vi "Pi_Python_REPL.vi"(11 "Pi IP Address":string="130.64.218.232") -> ()   [LabVIEW 2019]
panel:
  in  "Ctrl C":bool
  in  "Script":string="from pybricks import ev3brick as brick\nfrom pybricks.ev3devices import Motor, TouchSensor, ColorSensor,InfraredSensor, UltrasonicSensor, GyroSensor\n\nfrom pybricks.parameters import Port, Stop, Direction, Button, Color, Align\n\nfrom pybricks.tools import wait, StopWatch\n\nexample_motor = Motor (Port.A)"
  out "Console":string
  in  "Help Button":bool
  in  "Run DIrect":bool
  in  "Password":string="buddha"
  in  "Username":string="pi"
  out "SSH Success?":bool
  in  "Done":bool
  # "Get Labview running\n7. pip install paramiko  (SSH)\n8. Run this program\n9. hit ping to make sure it is there\n10. hit SSH In\n11. start python"
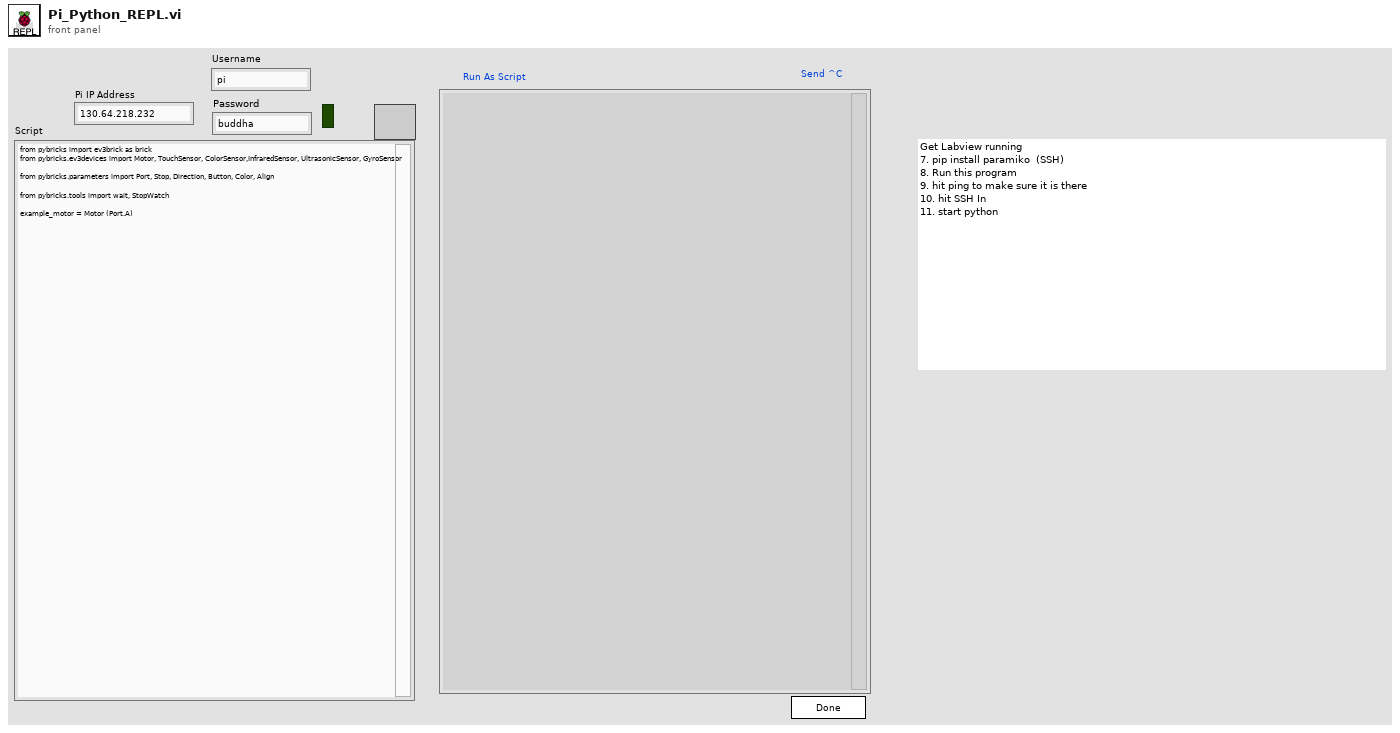
[diagram p1: front panel]
types:
  T1 = typedef "eventvkey.ctl" = enum16{"ASCII", "Enter", "Return", "Shift", "Ctrl", "Alt", "Cmd", "Opt", "Caps", "NumLock", "Clear", "Break", "Up", "Down", "Left", "Right", "Insert", "Delete", "Home", "End", "PageUp", "PageDown", "Escape", "Help", "Pause", "ScrollLock", "F1", "F2", "F3", "F4", "F5", "F6", "F7", "F8", "F9", "F10", "F11", "F12", "F13", "F14", "F15", "F16", "F17", "F18", "F19", "F20", "F21", "F22", "F23", "F24", "Play", "VolumeUp", "VolumeDown", "Mute", "Two Byte Char"}
  T2 = cluster{"Shift":bool, "Ctrl":bool, "Alt":bool, "Cmd":bool, "Opt":bool}
  T3 = cluster{"Char":i16, "VKey":T1, "ScanCode":i16, "Mods":cluster{"Num Pad":bool, "Menu Key":bool}, "PlatMods":cluster{"Shift":bool, "Ctrl":bool, "Alt":bool, "Cmd":bool, "Opt":bool}, "FocusObj":refnum<vi>}
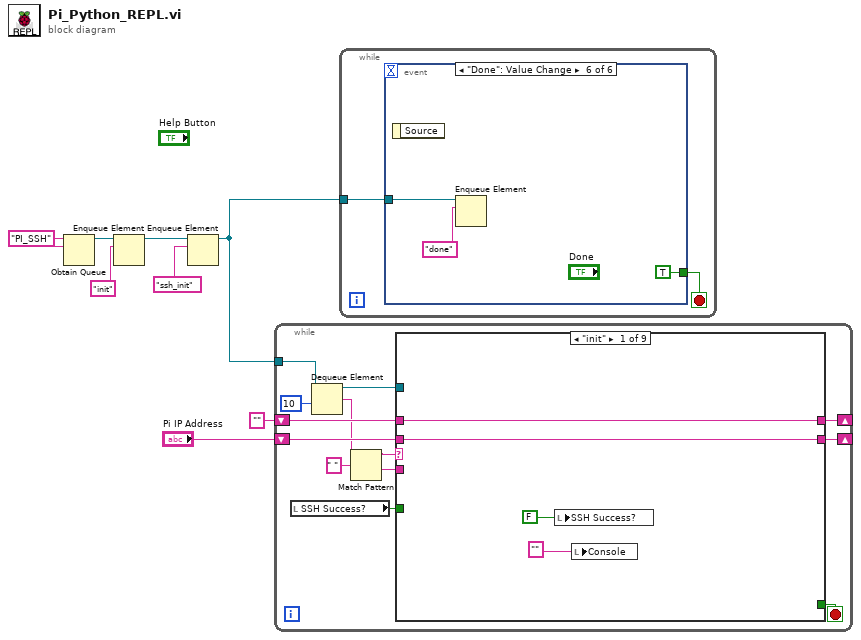
[diagram p0: block diagram]
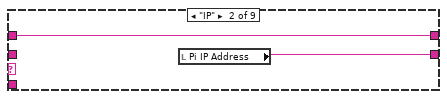
[diagram p2: hidden frame]
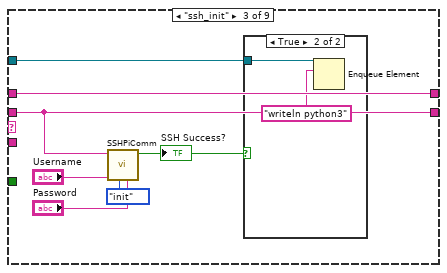
[diagram p3: hidden frame]
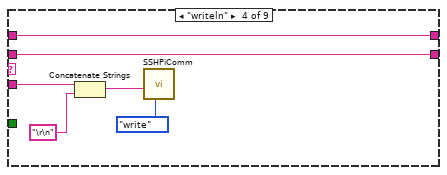
[diagram p5: hidden frame]
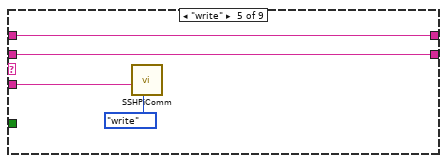
[diagram p6: hidden frame]
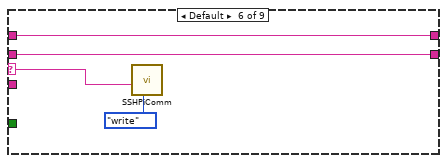
[diagram p7: hidden frame]
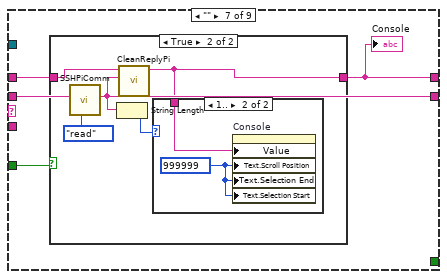
[diagram p8: hidden frame]
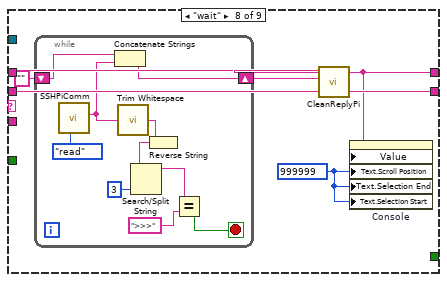
[diagram p11: hidden frame]
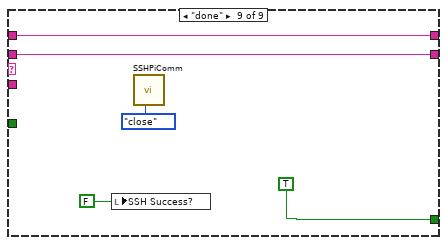
[diagram p12: hidden frame]
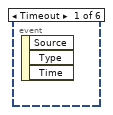
[diagram p13: hidden frame]
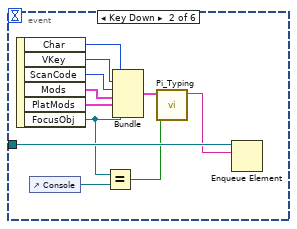
[diagram p14: hidden frame]
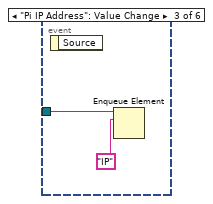
[diagram p15: hidden frame]
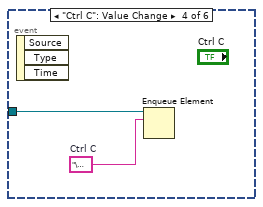
[diagram p16: hidden frame]
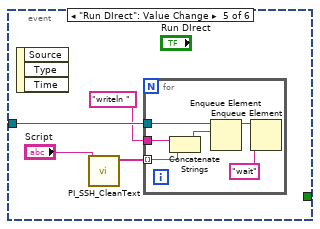
[diagram p17: hidden frame]
diagram:
  w6 = "PI_SSH" ("name (unnamed)")
  n1 = Obtain Queue(name (unnamed)=w6, element data type=w6) -> (queue out=w8:refnum<queue>)  [unwired: 3 in, 2 out]
  n2 = Enqueue Element(queue=w8, element="init") -> (queue out=w3:refnum<queue>)  [unwired: 2 in, 2 out]
  n3 = Enqueue Element(queue=w3, element="ssh_init") -> (queue out=w1:refnum<queue>)  [unwired: 2 in, 2 out]
  n4 = while {
    tunnel: w1 -> [w21]
    shift-right: [w18] -> _
    shift-left: "Pi IP Address" -> [w19]
    shift-right: [w16] -> _
    shift-left: "" -> [w17]
    stop <- w20 stop-if-true
    n5 = local read "SSH Success?"() -> (w10:bool)
    n6 = Dequeue Element(queue=w21, timeout in ms (-1)=10) -> (queue out=w9:refnum<queue>, element=w13:string)  [unwired: 1 in, 2 out]
    n7 = Match Pattern(string=w13, regular expression=" ") -> (before substring=w12:string, after substring=w11:string)  [unwired: 1 in, 2 out]
    n8 = case shown="\"init\"" w12 {
      selector: w12 -> [_ _ _ _ _ w47 _ _ _]
      tunnel: [_ _ _ _ _ _ _ _ TRUE] -> w20
      tunnel: w19 -> [w25 _ w32 w41 w45 w49 w54 w68 w82]
      tunnel: [w25 w27 w32 w41 w45 w49 w54 w68 w82] -> w18
      tunnel: w17 -> [w24 w26 w34 w42 w46 w50 w53 w63 w81]
      tunnel: [w24 w26 w34 w42 w46 w50 w52 w64 w81] -> w16
      tunnel: w11 -> [_ _ _ w37 w43 _ _ _ _]
      tunnel: w10 -> [_ _ _ _ _ _ w51 _ _]
      tunnel: w9 -> [_ _ w28 _ _ _ _ _ _]
      frame "init" {
        n9 = local write "SSH Success?"(FALSE ("Success?")) -> ()
        n10 = local write "Console"("" ("element")) -> ()
      }
      frame "IP" {
        n11 = local read "Pi IP Address"() -> (w27:string)
      }
      frame "ssh_init" {
        n12 = call "SSHPiComm.vi"("password"="Password", "Task"=enum16{"init", "read", "write", "close"}."init", "Username"="Username", "EV3 IP Address"=w32) -> ("Connected?"=w29:bool)  [unwired: 6 in, 1 out]
        "SSH Success?" <- w29
        n13 = case shown="True" w29 {
          tunnel: w28 -> [_ w35]
          frame False {
          }
          frame True {
            n14 = Enqueue Element(queue=w35, element="writeln python3") -> ()  [unwired: 2 in, 3 out]
          }
        }
      }
      frame "writeln" {
        n15 = Concatenate Strings(w37, "\r\n" ("regular expression")) -> (w38:string)
        n16 = call "SSHPiComm.vi"("Task"=enum16{"init", "read", "write", "close"}."write", "Text to write"=w38) -> ()  [unwired: 8 in, 2 out]
      }
      frame "write" {
        n17 = call "SSHPiComm.vi"("Task"=enum16{"init", "read", "write", "close"}."write", "Text to write"=w43) -> ()  [unwired: 8 in, 2 out]
      }
      frame Default {
        n18 = call "SSHPiComm.vi"("Task"=enum16{"init", "read", "write", "close"}."write", "Text to write"=w47) -> ()  [unwired: 8 in, 2 out]
      }
      frame "" {
        n19 = case shown="True" w51 {
          tunnel: w53 -> [w55 w60]
          tunnel: [w55 w56] -> w52
          frame False {
          }
          frame True {
            n20 = call "SSHPiComm.vi"("Task"=enum16{"init", "read", "write", "close"}."read") -> ("text read"=w58:string)  [unwired: 9 in, 1 out]
            n21 = String Length(string=w58) -> (length=w57:i32)
            n22 = call "CleanReplyPi.vi"("text read"=w58, "Console in"=w60) -> ("String out"=w56:string)  [unwired: 9 in]
            n23 = case shown="1.." w57 {
              tunnel: w56 -> [_ w61]
              frame 0, Default {
              }
              frame 1.. {
                w62 = u32 999999 ("Text.Scroll Position")
                n24 = property on="Console" class="Str"("Value"=w61, "Text.Scroll Position"=w62, "Text.Selection End"=w62, "Text.Selection Start"=w62) -> ()  [unwired: 2 in, 2 out]
              }
            }
          }
        }
        "Console" <- w52
      }
      frame "wait" {
        w65 = u32 999999 ("Text.Scroll Position")
        n25 = while {
          shift-right: [w76] -> w67
          shift-left: "" -> [w77]
          stop <- w69 stop-if-true
          n26 = call "SSHPiComm.vi"("Task"=enum16{"init", "read", "write", "close"}."read") -> ("text read"=w70:string)  [unwired: 9 in, 1 out]
          n27 = Concatenate Strings(w77, w70) -> (w76:string)
          n28 = call <vilib>:"Trim Whitespace.vi"("string"=w70) -> ("trimmed string"=w75:string)  [unwired: 1 in]
          n29 = Reverse String(1:w75) -> (0:w74:string)
          n30 = Search/Split String(string=w74, offset (0)=3) -> (substring before match=w71:string)  [unwired: 1 in, 2 out]
          n31 = Equal?(x=w71, y=">>>") -> (x = y?=w69:bool)
        }
        n32 = call "CleanReplyPi.vi"("text read"=w67, "Console in"=w63) -> ("String out"=w64:string)  [unwired: 9 in]
        n33 = property on="Console" class="Str"("Value"=w64, "Text.Scroll Position"=w65, "Text.Selection End"=w65, "Text.Selection Start"=w65) -> ()  [unwired: 2 in, 2 out]
      }
      frame "done" {
        n34 = local write "SSH Success?"(FALSE ("Success?")) -> ()
        n35 = call "SSHPiComm.vi"("Task"=enum16{"init", "read", "write", "close"}."close") -> ()  [unwired: 9 in, 2 out]
      }
    }
  }
  n36 = while {
    tunnel: w1 -> [w85]
    stop <- w84 stop-if-true
    n37 = event shown="[5] \"Done\": Value Change" {
      selector: _ -> [_ _ _ _ _ _]
      dyn-events: _ -> [_ _ _ _ _ _]
      timeout: _ -> [_ _ _ _ _ _]
      tunnel: w85 -> [_ w96 w97 w99 w104 w112]
      tunnel: [_ _ _ _ _ TRUE ("Done")] -> w84
      event Timeout {
        n38 = event-data() -> ()  [unwired: 1 in, 3 out]
      }
      event Key Down {
        n39 = event-data() -> ("Char"=w95:i16, "VKey"=w94:T1, "ScanCode"=w93:i16, "Mods"=w92:cluster{"Num Pad":bool, "Menu Key":bool}, "PlatMods"=w91:T2, "FocusObj"=w87:refnum<vi>)  [unwired: 1 in]
        n40 = control-ref of="Console"() -> (w88:refnum<vi>)
        n41 = Equal?(x=w87, y=w88) -> (x = y?=w86:bool)
        n42 = Bundle("Char"=w95, "VKey"=w94, "ScanCode"=w93, "Mods"=w92, "PlatMods"=w91, "FocusObj"=w87) -> (w90:T3)  [unwired: 1 in]
        n43 = call "Pi_Typing.vi"("Update"=w86, "Cluster"=w90) -> ("string"=w89:string)  [unwired: 7 in, 2 out]
        n44 = Enqueue Element(queue=w96, element=w89) -> ()  [unwired: 2 in, 3 out]
      }
      event "Pi IP Address": Value Change {
        n45 = event-data() -> ()  [unwired: 1 in, 1 out]
        n46 = Enqueue Element(queue=w97, element="IP") -> ()  [unwired: 2 in, 3 out]
      }
      event "Ctrl C": Value Change {
        w100 = "\u0003"  # Ctrl C
        n47 = event-data() -> ()  [unwired: 1 in, 3 out]
        n48 = Enqueue Element(queue=w99, element=w100) -> ()  [unwired: 2 in, 3 out]
      }
      event "Run DIrect": Value Change {
        n49 = event-data() -> ()  [unwired: 1 in, 3 out]
        n50 = call "PI_SSH_CleanText.vi"("Script"="Script") -> ("Array"=w102:string[])  [unwired: 10 in]
        n51 = for {
          tunnel: w104 -> [w110]
          tunnel: w102 -> [w109] mode=indexing
          tunnel: "writeln " ("format string") -> [w108]
          n52 = Concatenate Strings(w108, w109) -> (w107:string)
          n53 = Enqueue Element(queue=w110, element=w107) -> (queue out=w106:refnum<queue>)  [unwired: 2 in, 2 out]
          n54 = Enqueue Element(queue=w106, element="wait" ("format string")) -> ()  [unwired: 2 in, 3 out]
        }
      }
      event "Done": Value Change {
        n55 = event-data() -> ()  [unwired: 1 in, 1 out]
        n56 = Enqueue Element(queue=w112, element="done") -> ()  [unwired: 2 in, 3 out]
      }
    }
  }
